vi "get Rx Packet Error.vi"(10 "error":u8, 11 "protocol_version":i32) -> (3 "function return":string)   [LabVIEW 2021, in "dxl_x86_c.lvlib"]
doc: "WINDECLSPEC const char *getRxPacketError (int protocol_version, uint8_t error);"
uses:
  dxl_x86_c.lvlib
  dxl_x86_c.dll
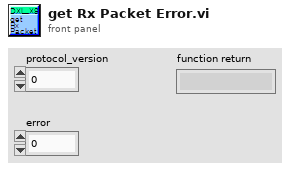
[diagram p1: front panel]
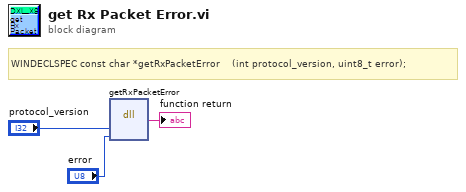
[diagram p0: block diagram]
diagram:
  # "WINDECLSPEC const char *getRxPacketError    (int protocol_version, uint8_t error);"
  n1 = dll-call lib="C:/Users/ashek/Desktop/ashekim/ws/DynamixelSDK/labview/labview/dxl_x86_c.*" fn="getRxPacketError"("protocol_version"="protocol_version", "error"="error") -> (→"function return":string)  [unwired: 5 in, 2 out]
